vi "Create SubVI.vi"(0 "Diagram in":refnum<vi>, 1 "VI Reference":refnum<vi>, 2 "location (0, 0)":T1, 5 "Input Names":string[](array[string]), 7 "Inputs":refnum<vi>[](array[refnum]), 9 "Output Names":string[](array[string]), 11 "error in (no error)":errorcluster) -> (4 "Diagram out":refnum<vi>, 6 "Outputs":refnum<vi>[](array[refnum]), 15 "error out":errorcluster)   [LabVIEW 2015, in "Scripting.lvlib"]
doc: "Creates a SubVI at <B>location</B> on <B>Diagram in</B>.\n\n<B>VI Reference</B> is a reference to the VI to be created.\n\n<B>Input Names</B> are the names of the input terminals to be wired on the created SubVI.\n\n<B>Inputs</B> are the terminals to wire to input terminals of the created SubVI.\n\n<B>Output Names</B> are the names of the needed output terminals of the created SubVI.\n\n<B>Outputs</B> are the selected output terminals of the created SubVI."
uses:
  Scripting.lvlib
  <vilib>/Utility/miscctls.llb/LVPointTypeDef.ctl
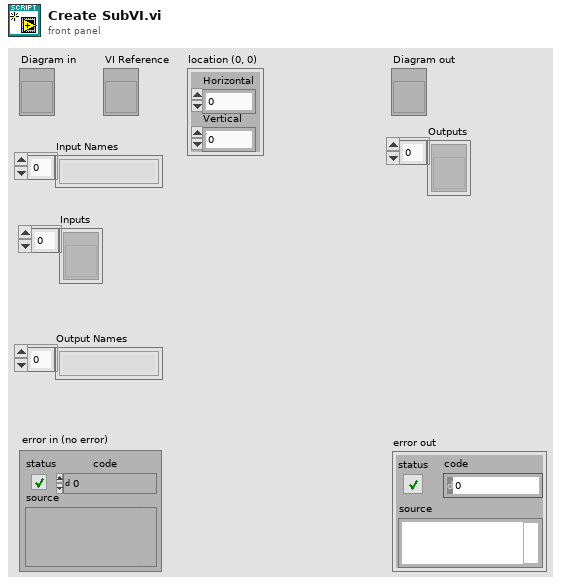
[diagram p1: front panel]
types:
  T1 = typedef "LVPointTypeDef.ctl" = cluster{"Horizontal":i16, "Vertical":i16}
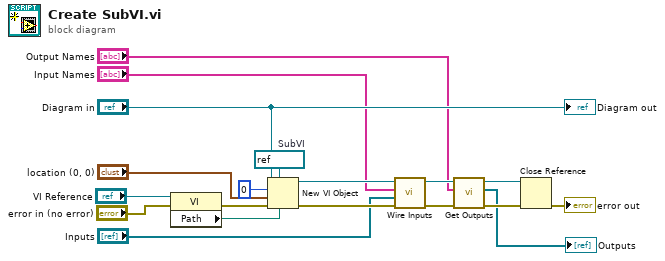
[diagram p0: block diagram]
diagram:
  w17 = refnum<vi> refnum  # SubVI
  n1 = property class="VI"(reference="VI Reference", error in="error in (no error)") -> (error out=w1:errorcluster, "Path"=w3:path)  [unwired: 1 out]
  n2 = New VI Object(vi object class=w17, owner refnum="Diagram in", style=0, position/next to="location (0, 0)", 6:w3, 8:w1) -> (object refnum=w11:refnum<vi>, 0:w9:errorcluster)  [unwired: 2 in]
  n3 = call "Wire Inputs.vi"("error in (no error)"=w9, "Inputs"="Inputs", "Names"="Input Names", "Node in"=w11) -> ("error out"=w13:errorcluster, "Node out"=w15:refnum<vi>)  [unwired: 6 in]
  n4 = call "Get Outputs.vi"("error in (no error)"=w13, "Names"="Output Names", "Node in"=w15) -> ("error out"=w14:errorcluster, "Outputs"=→"Outputs":refnum<vi>[], "Node out"=w8:refnum<vi>)  [unwired: 6 in]
  n5 = Close Reference(reference=w8, error in (no error)=w14) -> (error out=→"error out":errorcluster)
  "Diagram out" <- "Diagram in"
